vi "ScrapCode.vi"() -> ()   [LabVIEW 2012]
uses:
  <vilib>/FPGAPlugInAG/PCIe-7841R/niLvFpga_Open_PCIe-7841R.vi
  <vilib>/rvi/interface/common/dynamic/niFpgaDynamicAddResources.vi
  <vilib>/Utility/error.llb/Error Cluster From Error Code.vi
  <vilib>/rvi/errors/niLvFpgaAdjustHostInterfaceError.vi
  <vilib>/FPGAPlugInAG/Dynamic/niLvFpga_Close_Dynamic.vi
  <vilib>/rvi/interface/nirviOpenFPGA/nirviOpenFPGA.xnode
  FPGA Bitfiles/OptogeneticsTabl_FPGATarget_OpticsIO(FPGA)_9A6V+shJCSE.lvbitx
  OpticsIO (FPGA).vi
  <vilib>/rvi/interface/nirviReadWriteControl/nirviReadWriteControl.xnode
  <vilib>/rvi/interface/nirviCloseFPGA/nirviCloseFPGA.xnode
  <vilib>/rvi/interface/Simulation/niFpgaSimulationCallBeginRW.vi
  NiFpgaLv.dll
panel:
  in  "Frequency (Hz) A06":dbl=1000.0
  in  "Frequency (Hz) A07":dbl=1000.0
  in  "Continous A07":bool
  out "Connector0/AI6":i16(slide) scale=0.0..16384.0
  out "Connector0/AI6-val":i16
  out "Connector0/AI7":i16(slide) scale=0.0..16384.0
  out "Connector0/AI7-val":i16
  out "PWM Params A07":T1={"Pulse Length (Ticks)"=4294967295, "Pulse Period (Ticks)"=4294967295, "Ao (Int)"=0, "Seq 1 (High)"=TRUE, "Seq 2 (Low)"=TRUE}
  in  "stop":bool
  out "PWM Params A06":T1={"Pulse Length (Ticks)"=4294967295, "Pulse Period (Ticks)"=4294967295, "Ao (Int)"=0, "Seq 1 (High)"=TRUE, "Seq 2 (Low)"=TRUE}
  out "Transmission 2":dbl
  out "Transmission":dbl
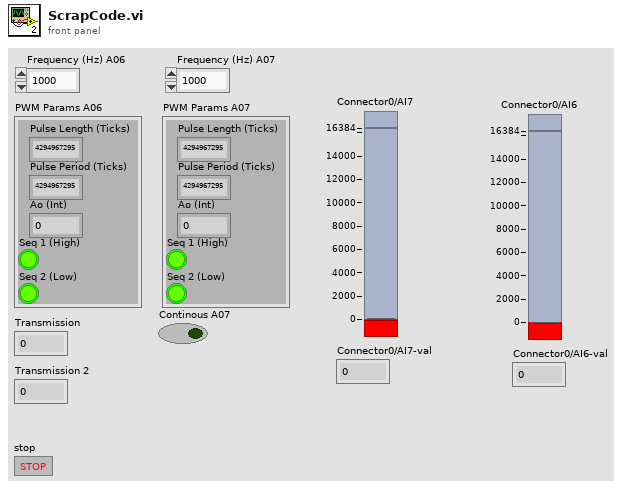
[diagram p1: front panel]
types:
  T1 = cluster{"Pulse Length (Ticks)":u32, "Pulse Period (Ticks)":u32, "Ao (Int)":i32, "Seq 1 (High)":bool, "Seq 2 (Low)":bool}
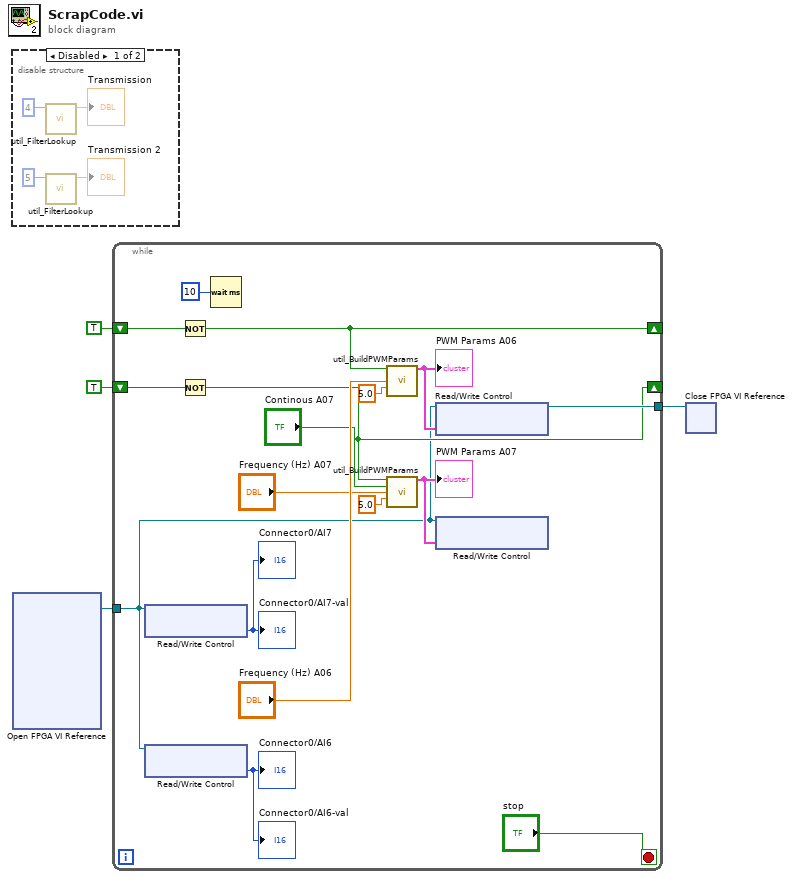
[diagram p0: block diagram]
diagram:
  n1 = disable-structure shown="Disabled" {
    frame Disabled {
      n2 = call "util_FilterLookup.vi"("Serial Port"=4) -> ("Transmission"=→"Transmission":dbl)  [unwired: 10 in]
      n3 = call "util_FilterLookup.vi"("Serial Port"=5) -> ("Transmission"=→"Transmission 2":dbl)  [unwired: 10 in]
    }
    frame Enabled {
    }
  }
  n4 = xnode "Open FPGA VI Reference"() -> ("FPGA VI Reference Out"=w3:refnum<k20>)  [unwired: 2 in, 1 out]
  n5 = while {
    tunnel: w3 -> [w11]
    tunnel: [w24] -> w4
    shift-right: [w20] -> _
    shift-left: TRUE -> [w21]
    shift-right: [w14] -> _
    shift-left: TRUE -> [w15]
    stop <- "stop" stop-if-true
    n6 = xnode "Read/Write Control"("FPGA VI Reference In"=w11) -> ("Connector0/AI7"=→"Connector0/AI7-val" →"Connector0/AI7":i16)  [unwired: 1 in, 2 out]
    n7 = xnode "Read/Write Control"("FPGA VI Reference In"=w11) -> ("Connector0/AI6"=→"Connector0/AI6-val" →"Connector0/AI6":i16)  [unwired: 1 in, 2 out]
    n8 = Not(x=w21) -> (.not. x?=w20:bool)
    n9 = Not(x=w15) -> (.not. x?=w14:bool)
    n10 = Wait (ms)(milliseconds to wait=u32 10) -> ()  [unwired: 1 out]
    n11 = call "util_BuildPWMParams.vi"("Burst"=w20, "Frequency (Hz)"="Frequency (Hz) A06", "Amplitude (V)"=5.0) -> ("PWM Params"=w25:T1)  [unwired: 12 in]
    "PWM Params A06" <- w25
    n12 = call "util_BuildPWMParams.vi"("Burst"=w14, "Continous"="Continous A07", "Frequency (Hz)"="Frequency (Hz) A07", "Amplitude (V)"=5.0) -> ("PWM Params"=w18:T1)  [unwired: 11 in]
    "PWM Params A07" <- w18
    n13 = xnode "Read/Write Control"("FPGA VI Reference In"=w11, "PWM Params A06"=w25) -> ("FPGA VI Reference Out"=w24:refnum<k20>)  [unwired: 1 in, 1 out]
    n14 = xnode "Read/Write Control"("FPGA VI Reference In"=w11, "PWM Params A07"=w18) -> ()  [unwired: 1 in, 2 out]
  }
  n15 = xnode "Close FPGA VI Reference"("FPGA VI Reference In"=w4) -> ()  [unwired: 1 in, 1 out]
